vi "Generator.Create AO waveforms.vi"(8 "error in (no error)":errorcluster, 10 "reset phase":bool, 11 "Generator in":refnum<class "Generator.lvclass">) -> (0 "error out":errorcluster, 2 "AO Array":waveform(dbl)[](array[waveform]), 3 "Generator out":refnum<class "Generator.lvclass">)   [LabVIEW 2019, in "Generator.lvclass"]
uses:
  Generator.lvclass
  <vilib>/measure/NI_MABase.lvlib
  <vilib>/Waveform/WDTOps.llb/WDT Append Waveforms DBL.vi
  Instrument.DAQ/Typedefs/AO.Channel.Function--Enum.ctl
  Instrument.DAQ/Instrument.DAQ.lvclass
  Instrument.DAQ/Typedefs/AO.Channel--Cluster.ctl
  Instrument.DAQ/Typedefs/AO.Channel--Cluster--Array.ctl
panel:
  in  "Tab Control":enum32{"Page 1", "Graphs"}(tab)
  out "Channels: AO":T1 {"Phase" format="%.2g"; "Frequency" min=0.0001 max=10000.0 format="%.2g"; "Offset" format="%5.2p"; "Amplitude" min=0.0 max=10.0 format="%5.2p"}
  in  "y":dbl format="%#_13g"
  out "Waveform Graph":waveform(dbl)[](graph)
  out "Waveform Chart":dbl[][](graph)
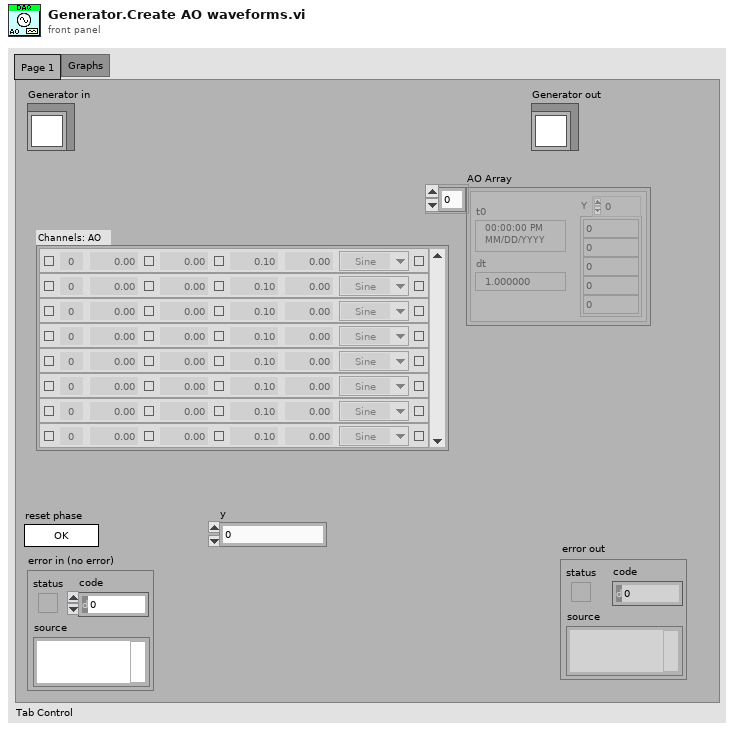
[diagram p1: front panel]
types:
  T1 = typedef "Instrument.Lockin.lvlib/Instrument.DAQ.lvclass/AO.Channel--Cluster--Array.ctl" = T2[]
  T2 = typedef "Instrument.Lockin.lvlib/Instrument.DAQ.lvclass/AO.Channel--Cluster.ctl" = cluster{"Enable?":bool, "Channel":i32, "Amplitude":dbl, "Offset":dbl, "Frequency":dbl, "Phase":dbl, "Function":T3, "Sweeping?":bool, "Limit AC":bool, "Limit DC?":bool}
  T3 = typedef "Instrument.Lockin.lvlib/Instrument.DAQ.lvclass/AO.Channel.Function--Enum.ctl" = enum16{"Sine", "Triangle", "Square"}
  T4 = typedef "Instrument.Lockin.lvlib/Instrument.DAQ.lvclass/REF.Channel--Cluster--Array.ctl" = T5[]
  T5 = typedef "Instrument.Lockin.lvlib/Instrument.DAQ.lvclass/REF.Channel--Cluster.ctl" = cluster{"Enable?":bool, "Channel":i32, "Frequency":dbl, "Phase":dbl, "TC":dbl, "Roll-Off":i32}
  T6 = enum16{"Sine Wave", "Triangle Wave", "Square Wave", "Sawtooth Wave"}
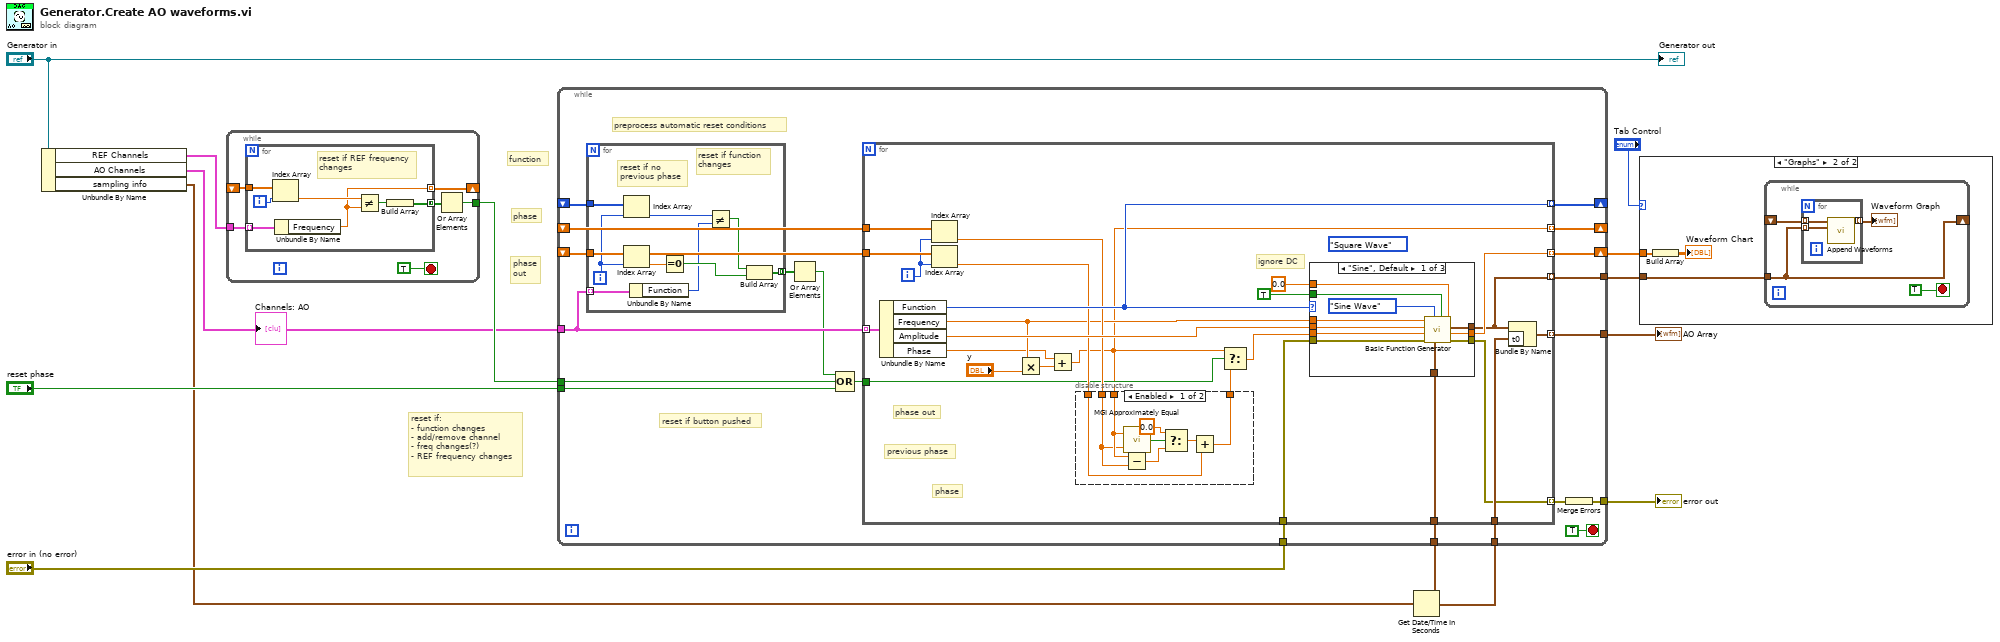
[diagram p0: block diagram]
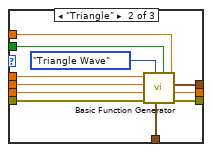
[diagram p3: hidden frame]
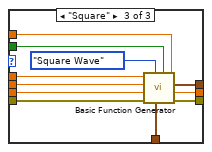
[diagram p4: hidden frame]
diagram:
  # "phase"
  # "function"
  # "phase\nout"
  # "reset if:\n- function changes\n- add/remove channel\n- freq changes(?)\n- REF frequency changes"
  n1 = Unbundle By Name("Generator in") -> ("REF Channels"=w2:T4, "AO Channels"=w3:T1, "sampling info"=w1:cluster{"Fs":dbl, "#s":dbl})
  "Channels: AO" <- w3
  n2 = while {
    tunnel: w2 -> [w19]
    shift-right: [w18] -> _
    shift-left: _ -> [w17]
    tunnel: [w14] -> w8
    stop <- TRUE stop-if-true
    n3 = for {
      tunnel: w19 -> [w21] mode=indexing
      tunnel: w17 -> [w25]
      tunnel: [w22] -> w15 mode=concatenating
      tunnel: [w20] -> w18 mode=indexing
      i -> [w26]
      # "reset if REF frequency\nchanges"
      n4 = Index Array(array=w25, index=w26) -> (element=w24:dbl)
      n5 = Unbundle By Name(w21) -> ("Frequency"=w20:dbl)
      n6 = Not Equal?(x=w24, y=w20) -> (x != y?=w23:bool)
      n7 = Build Array(w23) -> (w22:bool[])
    }
    n8 = Or Array Elements(Boolean array=w15) -> (logical OR=w14:bool)
  }
  n9 = Get Date/Time In Seconds() -> (seconds since 1Jan1904=w12:timestamp)
  n10 = while {
    tunnel: w1 -> [w46]
    tunnel: [w45] -> w10
    shift-right: [w43] -> w9
    shift-left: _ -> [w32]
    tunnel: w12 -> [w42]
    tunnel: "reset phase" -> [w36]
    tunnel: "error in (no error)" -> [w41]
    tunnel: [w39] -> w11
    tunnel: w3 -> [w38]
    shift-right: [w34] -> _
    shift-left: _ -> [w33]
    shift-right: [w31] -> _
    shift-left: _ -> [w30]
    tunnel: w8 -> [w29]
    tunnel: [w28] -> w7
    stop <- TRUE stop-if-true
    # "reset if button pushed"
    # "preprocess automatic reset conditions"
    n11 = for {
      tunnel: w38 -> [w48] mode=indexing
      tunnel: w32 -> [w55]
      tunnel: w33 -> [w54]
      tunnel: [w49] -> w37 mode=concatenating
      i -> [w56]
      # "reset if function\nchanges"
      # "reset if no\nprevious phase"
      n12 = Index Array(array=w54, index=w56) -> (element=w52:T3)
      n13 = Index Array(array=w55, index=w56) -> (element=w53:dbl)
      n14 = Unbundle By Name(w48) -> ("Function"=w47:T3)
      n15 = Equal To 0?(x=w53) -> (x = 0?=w50:bool)
      n16 = Not Equal?(x=w52, y=w47) -> (x != y?=w51:bool)
      n17 = Build Array(w51, w50) -> (w49:bool[])
    }
    n18 = Or Array Elements(Boolean array=w37) -> (logical OR=w27:bool)
    n19 = Compound Arithmetic op=OR(w27, w29, w36) -> (w35:bool)
    n20 = for {
      tunnel: [w79] -> w45 mode=indexing
      tunnel: w46 -> [w77]
      tunnel: [w63] -> w43 mode=indexing
      tunnel: w42 -> [w81]
      tunnel: w41 -> [w75]
      tunnel: [w78] -> w40 mode=indexing
      tunnel: w38 -> [w74] mode=indexing
      tunnel: w35 -> [w64]
      tunnel: [w72] -> w34 mode=indexing
      tunnel: w32 -> [w71]
      tunnel: [w57] -> w31 mode=indexing
      tunnel: w30 -> [w67]
      tunnel: [w62] -> w28 mode=indexing
      i -> [w70]
      (unwired) T6."Square Wave" ("signal type")
      # "previous phase"
      # "phase"
      # "phase out"
      # "ignore DC"
      n21 = Unbundle By Name(w74) -> ("Function"=w72:T3, "Frequency"=w59:dbl, "Amplitude"=w73:dbl, "Phase"=w58:dbl)
      n22 = Index Array(array=w67, index=w70) -> (element=w68:dbl)
      n23 = Index Array(array=w71, index=w70) -> (element=w69:dbl)
      n24 = Multiply(x=w59, y="y") -> (x*y=w60:dbl)
      n25 = Add(x=w58, y=w60) -> (x+y=w57:dbl)
      n26 = disable-structure shown="Enabled" {
        disable-tunnel: w57 -> [w88 _]
        disable-tunnel: w68 -> [w87 _]
        disable-tunnel: w69 -> [w82 w90]
        disable-tunnel: [w85 w90] -> w66
        frame Enabled {
          n27 = call <userlib>:"MGI Approximately Equal.vi"("Numeric 2"=w87, "Numeric 1"=w88) -> ("approx = ?"=w86:bool)
          n28 = Subtract(x=w88, y=w87) -> (x-y=w84:dbl)
          n29 = Select(t=0.0, s=w86, f=w84) -> (s? t:f=w83:dbl)
          n30 = Add(x=w83, y=w82) -> (x+y=w85:dbl)
        }
        frame Disabled {
        }
      }
      n31 = Select(t=w57, s=w64, f=w66) -> (s? t:f=w65:dbl)
      n32 = case shown="\"Sine\", Default" w72 {
        tunnel: w59 -> [w101 w112 w123]
        tunnel: 0.0 ("AO DC") -> [w100 w111 w122]
        tunnel: [w99 w110 w121] -> w62
        tunnel: TRUE ("reset signal") -> [w91 w102 w113]
        tunnel: w75 -> [w98 w109 w120]
        tunnel: [w97 w108 w119] -> w78
        tunnel: [w96 w107 w118] -> w63
        tunnel: w73 -> [w95 w106 w117]
        tunnel: w65 -> [w94 w105 w116]
        tunnel: w77 -> [w93 w104 w115]
        frame "Sine", Default {
          n33 = call <vilib>:"Basic Function Generator.vi"("offset"=w100, "reset signal"=w91, "sampling info"=w93, "signal type"=T6."Sine Wave", "error in (no error)"=w98, "phase"=w94, "amplitude"=w95, "frequency"=w101) -> ("error out"=w97:errorcluster, "phase out"=w96:dbl, "signal out"=w99:waveform(dbl))  [unwired: 1 in]
        }
        frame "Triangle" {
          n34 = call <vilib>:"Basic Function Generator.vi"("offset"=w111, "reset signal"=w102, "sampling info"=w104, "signal type"=T6."Triangle Wave", "error in (no error)"=w109, "phase"=w105, "amplitude"=w106, "frequency"=w112) -> ("error out"=w108:errorcluster, "phase out"=w107:dbl, "signal out"=w110:waveform(dbl))  [unwired: 1 in]
        }
        frame "Square" {
          n35 = call <vilib>:"Basic Function Generator.vi"("offset"=w122, "reset signal"=w113, "sampling info"=w115, "signal type"=T6."Square Wave", "error in (no error)"=w120, "phase"=w116, "amplitude"=w117, "frequency"=w123) -> ("error out"=w119:errorcluster, "phase out"=w118:dbl, "signal out"=w121:waveform(dbl))  [unwired: 1 in]
        }
      }
      n36 = Bundle By Name(cluster=w62, "t0"=w81) -> (w79:waveform(dbl))
    }
    n37 = Merge Errors(w40) -> (w39:errorcluster)
  }
  "AO Array" <- w10
  "error out" <- w11
  n38 = case shown="\"Graphs\"" "Tab Control" {
    tunnel: w7 -> [_ w124]
    tunnel: w9 -> [_ w125]
    frame Default {
    }
    frame "Graphs" {
      n39 = Build Array(w125) -> (→"Waveform Chart":dbl[][])
      n40 = while {
        shift-right: [w127] -> _
        shift-left: _ -> [w128]
        tunnel: w124 -> [w127]
        stop <- TRUE stop-if-true
        n41 = for {
          tunnel: [w133] -> w129 mode=indexing
          tunnel: w128 -> [w132] mode=indexing
          tunnel: w127 -> [w131] mode=indexing
          n42 = call-poly <vilib>:"Append Waveforms.vi"("waveform B"=w131, "waveform A"=w132) -> ("waveform out"=w133:waveform(dbl))  [unwired: 8 in, 1 out]
        }
        "Waveform Graph" <- w129
      }
    }
  }
  "Generator out" <- "Generator in"
